vi "ultrasonic_pid.vi"(0 "Setpoint":sgl, 1 "Time":u32, 2 "KF":sgl, 3 "Error":sgl, 5 "Input":sgl, 7 "KP":sgl, 9 "KI":dbl, 11 "KD":dbl, 12 "Previous Time":u32, 13 "Feed Forward":sgl, 14 "Accumulated Error":dbl) -> (4 "Output":dbl, 6 "Error":sgl, 10 "Current Time":dbl, 15 "Accumulated Error":dbl)   [LabVIEW 2016]
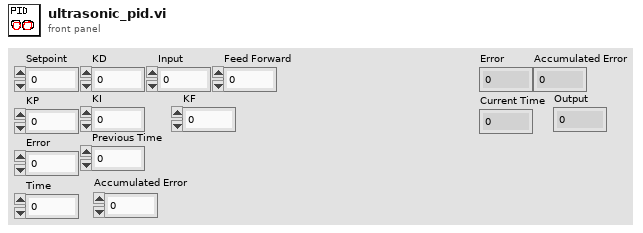
[diagram p1: front panel]
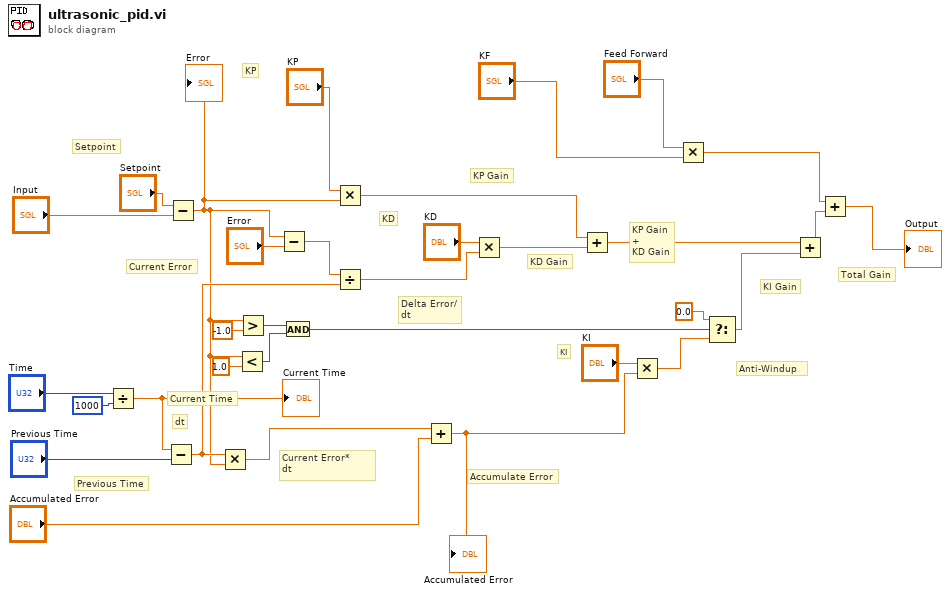
[diagram p0: block diagram]
diagram:
  # "Current Time"
  # "Anti-Windup"
  # "Previous Time"
  # "Total Gain"
  # "KD Gain"
  # "KP Gain\n+\nKD Gain"
  # "KI Gain"
  # "Current Error*\ndt"
  # "Accumulate Error"
  # "Delta Error/\ndt"
  # "Setpoint"
  # "KP Gain"
  # "dt"
  # "Current Error"
  # "KI"
  # "KD"
  # "KP"
  n1 = Divide(x="Time", y=u32 1000) -> (x/y=w9:dbl)
  "Current Time" <- w9
  n2 = Subtract(x=w9, y="Previous Time") -> (x-y=w29:dbl)
  n3 = Subtract(x="Setpoint", y="Input") -> (x-y=w19:sgl)
  "Error" <- w19
  n4 = Multiply(x=w29, y=w19) -> (x*y=w26:dbl)
  n5 = Less?(x=w19, y=sgl 1.0) -> (x < y?=w16:bool)
  n6 = Greater?(x=w19, y=sgl -1.0) -> (0:w20:bool)
  n7 = Subtract(x=w19, y="Error") -> (x-y=w33:sgl)
  n8 = And(x=w20, y=w16) -> (x .and. y?=w21:bool)
  n9 = Multiply(x="KP", y=w19) -> (x*y=w28:sgl)
  n10 = Divide(x=w33, y=w29) -> (x/y=w32:dbl)
  n11 = Add(x=w26, y="Accumulated Error") -> (x+y=w25:dbl)
  "Accumulated Error" <- w25
  n12 = Multiply(x="KD", y=w32) -> (x*y=w27:dbl)
  n13 = Add(x=w28, y=w27) -> (x+y=w31:dbl)
  n14 = Multiply(x="KI", y=w25) -> (x*y=w24:dbl)
  n15 = Multiply(x="Feed Forward", y="KF") -> (x*y=w3:sgl)
  n16 = Select(t=0.0, s=w21, f=w24) -> (s? t:f=w22:dbl)
  n17 = Add(x=w31, y=w22) -> (x+y=w2:dbl)
  n18 = Add(x=w3, y=w2) -> (x+y=→"Output":dbl)
